vi "VNS Frame.vi"() -> ()   [LabVIEW 2013]
uses:
  <vilib>/Analysis/1siggen.llb/Riffle Array (I32).vi
  <vilib>/Analysis/NI_AALBase.lvlib
  Classes/GanntChart.lvclass
panel:
  out "VNS Result":i32[](array[numeric])
  out "Best Chromosome":i32[](array[numeric])
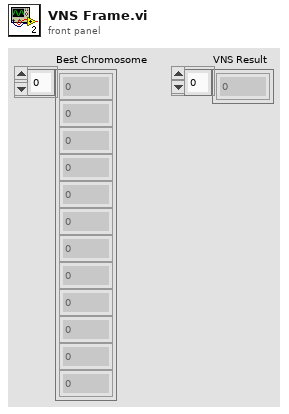
[diagram p1: front panel]
types:
  T1 = typedef "GanntChart_Element.ctl" = cluster{"Operation Number":i32, "Job Number":i32, "Start Time":i32, "Procesing Time":u16, "End Time":i32}
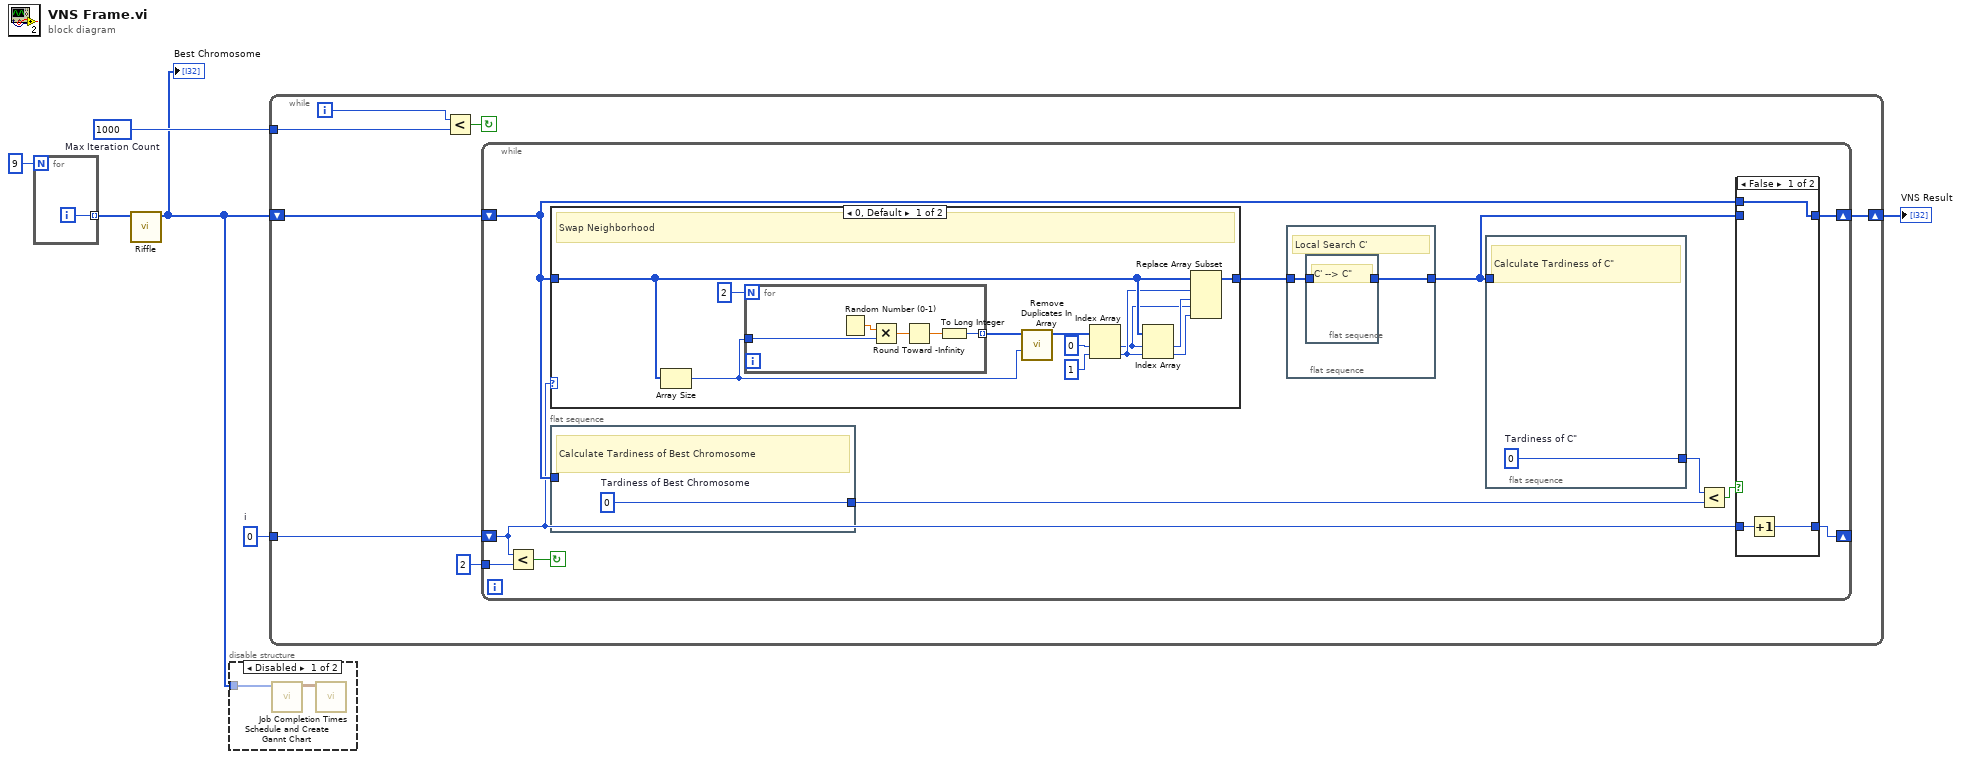
[diagram p0: block diagram]
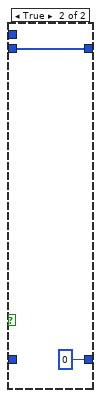
[diagram p3: hidden frame]
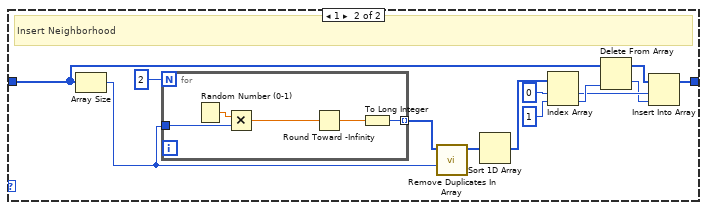
[diagram p4: hidden frame]
diagram:
  w3 = 0  # i
  w4 = 1000  # Max Iteration Count
  n1 = for {
    N: 9 -> [_]
    tunnel: [w7] -> w5 mode=indexing
    i -> [w7]
  }
  n2 = call-poly <vilib>:"Riffle.vi"("X"=w5) -> ("Riffled {X}"=w2:i32[])  [unwired: 8 in, 2 out]
  "Best Chromosome" <- w2
  n3 = disable-structure shown="Disabled" {
    disable-tunnel: w2 -> [w9 _]
    frame Disabled {
      n4 = call "Schedule and Create Gannt Chart.vi"("Schedule"=w9) -> ("Gannt Chart Out"=w8:T1[][])  [unwired: 9 in, 1 out]
      n5 = call "Job Completion Times.vi"("Gannt Chart In"=w8) -> ()  [unwired: 10 in, 1 out]
    }
    frame Enabled {
    }
  }
  n6 = while {
    tunnel: w4 -> [w16]
    tunnel: w3 -> [w13]
    shift-right: [w10] -> w1
    shift-left: w2 -> [w12]
    i -> [w11]
    stop <- w15 continue-if-true
    n7 = Less?(x=w11, y=w16) -> (x < y?=w15:bool)
    n8 = while {
      tunnel: 2 -> [w22]
      shift-right: [w21] -> _
      shift-left: w13 -> [w17]
      shift-right: [w20] -> w10
      shift-left: w12 -> [w19]
      stop <- w27 continue-if-true
      n9 = Less?(x=w17, y=w22) -> (x < y?=w27:bool)
      n10 = case shown="0, Default" w17 {
        tunnel: w19 -> [w43 w62]
        tunnel: [w38 w55] -> w26
        frame 0, Default {
          # "Swap Neighborhood"
          n11 = Array Size(array=w43) -> (size(s)=w47:i32)
          n12 = for {
            N: 2 -> [_]
            tunnel: w47 -> [w53]
            tunnel: [w50] -> w48 mode=indexing
            n13 = Random Number (0-1)() -> (number: 0 to 1=w54:dbl)
            n14 = Multiply(x=w54, y=w53) -> (x*y=w52:dbl)
            n15 = Round Toward -Infinity(1:w52) -> (0:w51:dbl)
            n16 = To Long Integer(number=w51) -> (32bit integer=w50:i32)
          }
          n17 = call "Remove Duplicates In Array.vi"("Max Index Bound"=w47, "Random Numbers Array"=w48) -> ("Random Numbers Array without Duplicates"=w46:i32[])  [unwired: 9 in]
          n18 = Index Array(array=w46, index #1=0 ("index"), index #2=1 ("index")) -> (element #1=w40:i32, element #2=w42:i32)
          n19 = Index Array(array=w43, index #1=w40, index #2=w42) -> (element #1=w41:i32, element #2=w39:i32)
          n20 = Replace Array Subset(array=w43, new element #1=w41, index #1=w42, new element #2=w39, index #2=w40) -> (w38:i32[])
        }
        frame 1 {
          # "Insert Neighborhood"
          n21 = Array Size(array=w62) -> (size(s)=w65:i32)
          n22 = for {
            N: 2 -> [_]
            tunnel: w65 -> [w71]
            tunnel: [w68] -> w66 mode=indexing
            n23 = Random Number (0-1)() -> (number: 0 to 1=w72:dbl)
            n24 = Multiply(x=w72, y=w71) -> (x*y=w70:dbl)
            n25 = Round Toward -Infinity(1:w70) -> (0:w69:dbl)
            n26 = To Long Integer(number=w69) -> (32bit integer=w68:i32)
          }
          n27 = call "Remove Duplicates In Array.vi"("Max Index Bound"=w65, "Random Numbers Array"=w66) -> ("Random Numbers Array without Duplicates"=w60:i32[])  [unwired: 9 in]
          n28 = Sort 1D Array(array=w60) -> (sorted array=w59:i32[])
          n29 = Index Array(array=w59, index #1=0 ("index"), index #2=1 ("index")) -> (element #1=w57:i32, element #2=w58:i32)
          n30 = Delete From Array(array=w62, index=w58) -> (deleted portion=w56:i32, array with subset deleted=w61:i32[])  [unwired: 1 in]
          n31 = Insert Into Array(array=w61, index=w57, new element=w56) -> (w55:i32[])
        }
      }
      n32 = flat-sequence {
        tunnel: w19 -> [_]
        tunnel: [w29] -> w24
        frame #0 {
          w29 = 0  # Tardiness of Best Chromosome
          # "Calculate Tardiness of Best Chromosome"
        }
      }
      n33 = flat-sequence {
        tunnel: w26 -> [w36]
        tunnel: [w35] -> w18
        frame #0 {
          # "Local Search C'"
          n34 = flat-sequence {
            tunnel: w36 -> [w37]
            tunnel: [w37] -> w35
            frame #0 {
              # "C' --> C\""
            }
          }
        }
      }
      n35 = flat-sequence {
        tunnel: w18 -> [_]
        tunnel: [w28] -> w25
        frame #0 {
          w28 = 0  # Tardiness of C"
          # "Calculate Tardiness of C\""
        }
      }
      n36 = Less?(x=w25, y=w24) -> (x < y?=w23:bool)
      n37 = case shown="False" w23 {
        tunnel: w17 -> [w31 _]
        tunnel: w18 -> [_ w33]
        tunnel: [w32 0] -> w21
        tunnel: [w30 w33] -> w20
        tunnel: w19 -> [w30 _]
        frame False {
          n38 = Increment(x=w31) -> (x+1=w32:i32)
        }
        frame True {
        }
      }
    }
  }
  "VNS Result" <- w1
